vi "Lavi_Ariel_soundboard.vi"() -> ()   [LabVIEW 2016]
uses:
  <vilib>/sound2/lvsound2.llb/Sound Data Format.ctl
  <vilib>/sound2/lvsound2.llb/Sampling Mode.ctl
  <vilib>/sound2/lvsound2.llb/Sound File Position.ctl
  <vilib>/sound2/lvsound2.llb/Sound File Write Open.vi
  <vilib>/sound2/lvsound2.llb/Sound Input Read (DBL).vi
  <vilib>/sound2/lvsound2.llb/Sound File Write (DBL).vi
  <vilib>/sound2/lvsound2.llb/Sound File Info (path).vi
  <vilib>/sound2/lvsound2.llb/Sound File Read Open.vi
  <vilib>/sound2/lvsound2.llb/Sound File Read (DBL).vi
  <vilib>/sound2/lvsound2.llb/Sound Output Set Volume (Single).vi
  <vilib>/sound2/lvsound2.llb/Sound Output Write (DBL).vi
  <vilib>/measure/maspectr.llb/FFT Power Spectrum and PSD for 1 Chan.vi
  <vilib>/measure/NI_MAPro.lvlib
panel:
  in  "Volume":dbl(knob)=100.0 scale=0.0..100.0
  in  "Record start":bool
  in  "Exit":bool
  in  "Menu":bool
  in  "STOP":bool
  in  "Play":bool
  out "f0":dbl
  out "df (increment)":dbl
  out "magnitude":dbl[](array[numeric])
  in  "Playback speed":dbl=1.0
  out "Waveform Graph 2":waveform(dbl)[](graph)
  in  "Upper Cut-Off (Hz)":dbl(slide)=400.0 caption="Upper Cut-Off" scale=20.0..20000.0
  in  "Lower Cut-Off (Hz)":dbl(slide)=100.0 caption="Lower Cut-Off" scale=20.0..20000.0
  in  "Filter enable":bool
  out "Save File path":path
  in  "Pause":bool
  out "Temporary Input File Path":path
  in  "output device ID":u32
  out "Waveform Graph":waveform(dbl)[](graph)
  in  "Record stop":bool
  in  "input device ID":u32
  # "Output Controls/Indicators"
  # "Input Controls/Indicators"
  # "Playback Controls"
  # "NOTE: The \"Menu\" button always\nreturns the user to the last main \nmenu. The \"Exit\" button always\ncauses the VI to stop and close."
  # "Fourier Analysis"
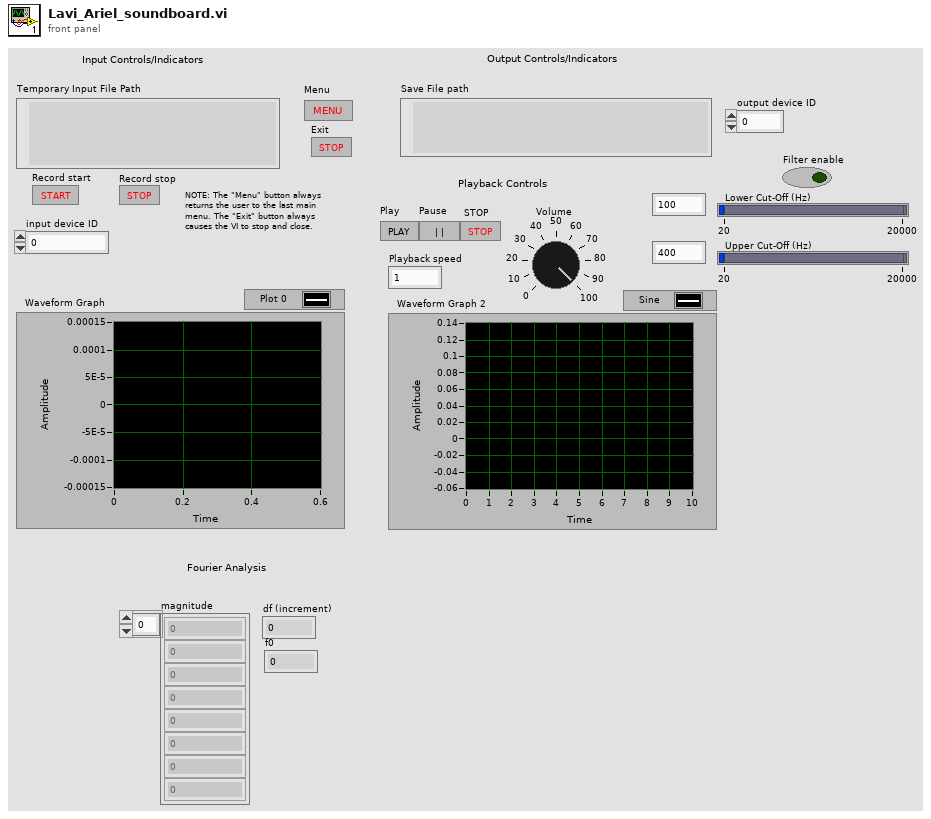
[diagram p1: front panel]
types:
  T1 = typedef "Sampling Mode.ctl" = i32
  T2 = typedef "Sound Data Format.ctl" = cluster{"sample rate (S/s)":dbl, "number of channels":i32, "bits per sample":i32}
  T3 = typedef "Sound File Refnum.ctl" = refnum<file>
  T4 = typedef "Sound Input Task ID.ctl" = u32
  T5 = cluster{dbl, "number of channels":i32, "bits per sample":i32}
  T6 = typedef "Sound Output Task ID.ctl" = u32
  T7 = typedef "Sound File Position.ctl" = u16
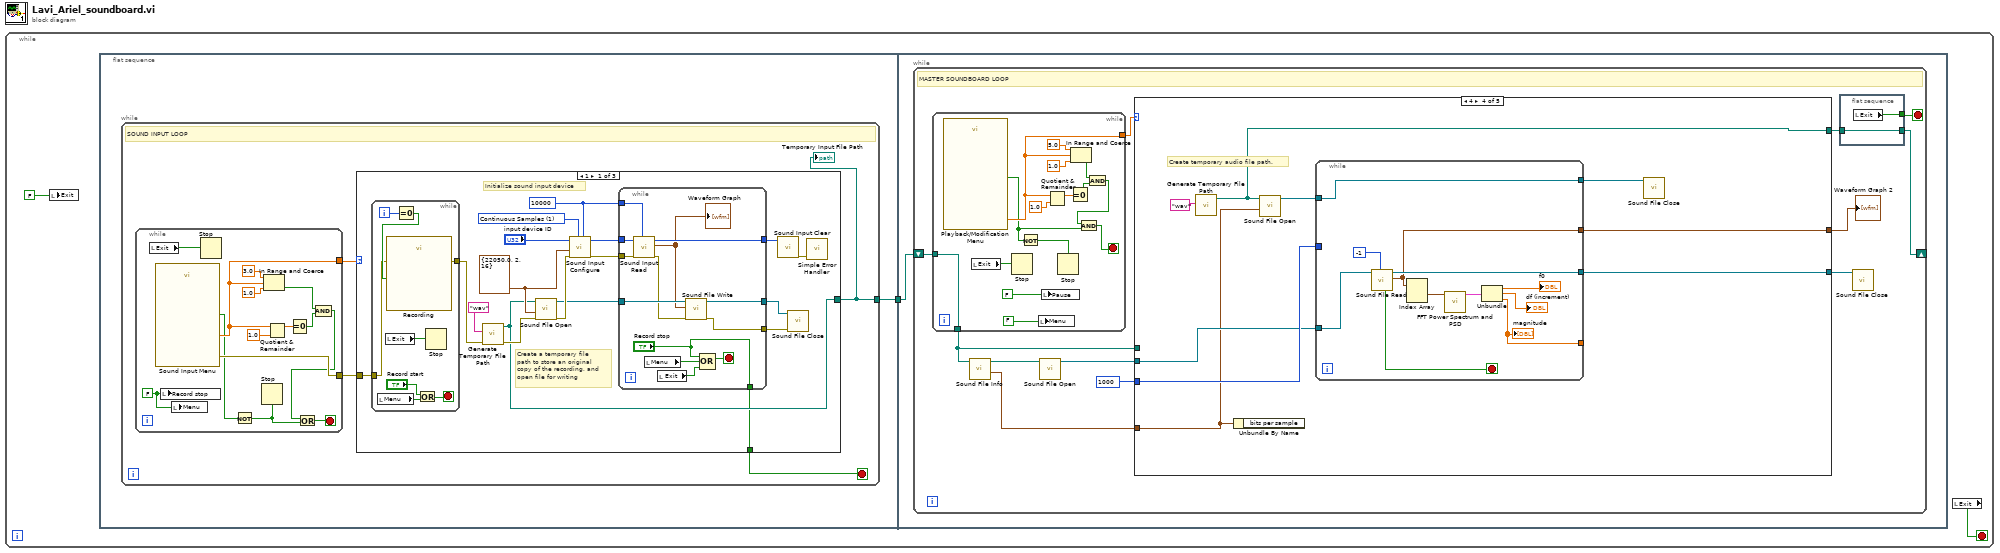
[diagram p0: block diagram]
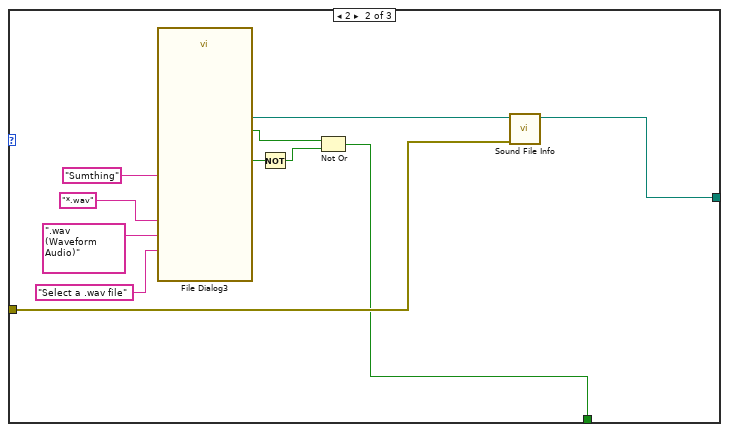
[diagram p2: hidden frame]
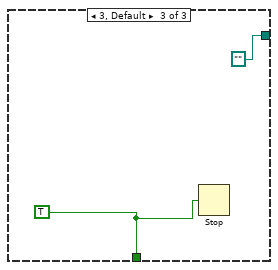
[diagram p3: hidden frame]
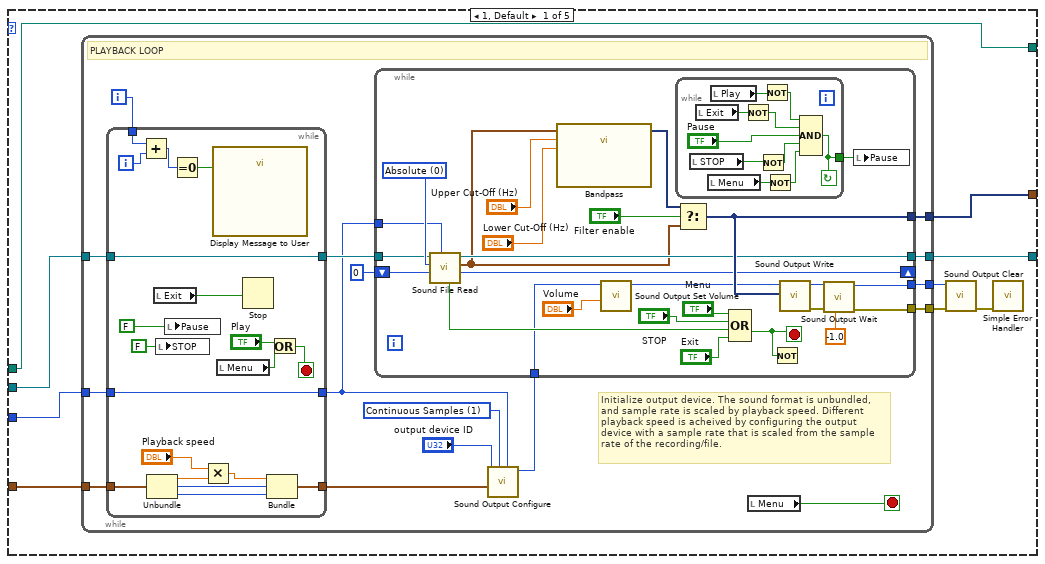
[diagram p4: hidden frame]
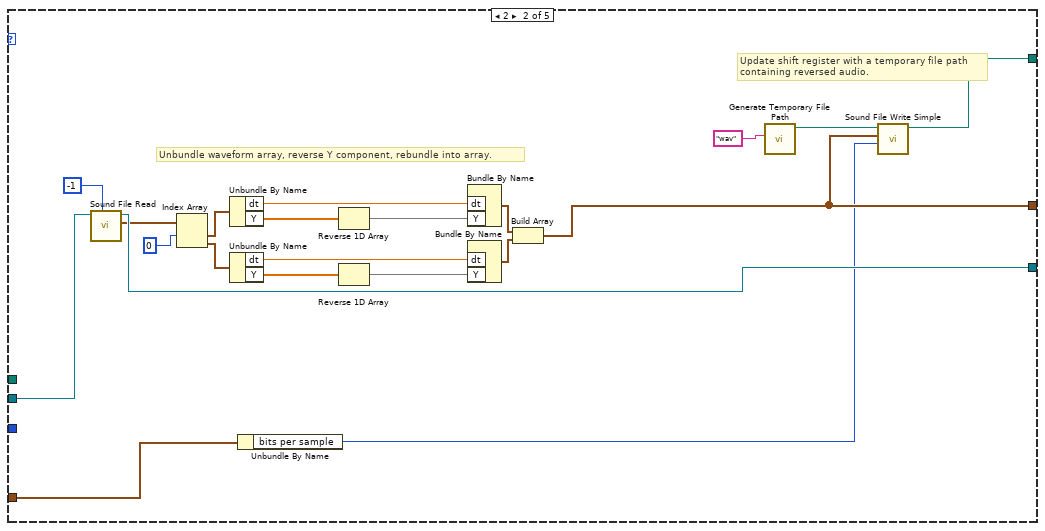
[diagram p5: hidden frame]
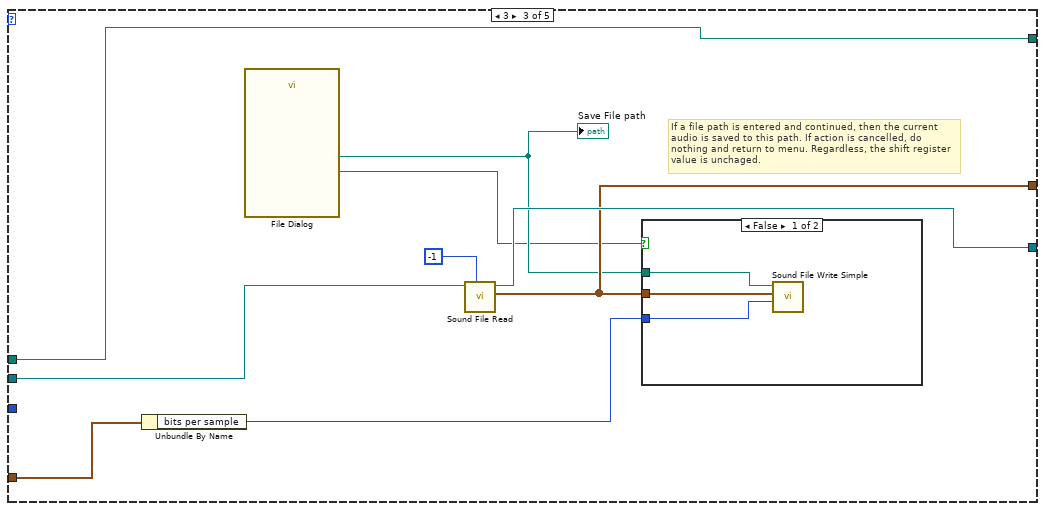
[diagram p6: hidden frame]
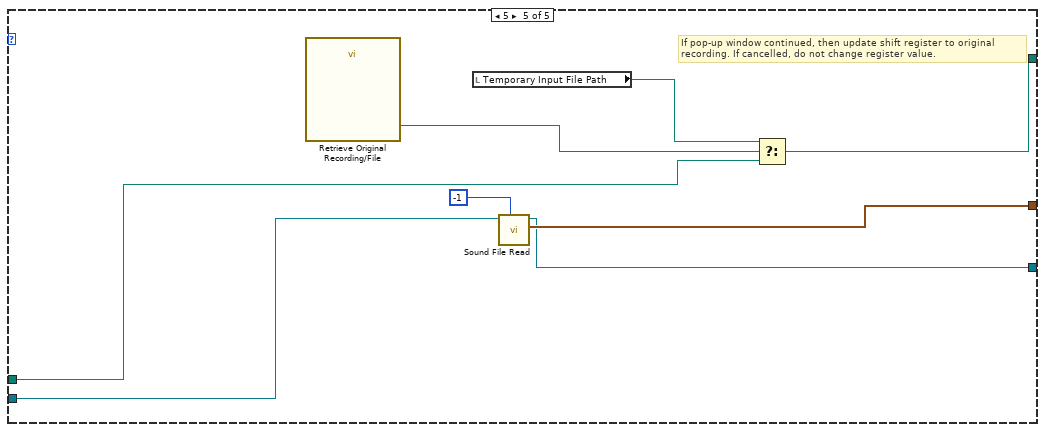
[diagram p8: hidden frame]
diagram:
  n1 = while {
    stop <- w1 stop-if-true
    n2 = local write "Exit"(FALSE) -> ()
    n3 = flat-sequence {
      tunnel: [w4] -> w3
      tunnel: w3 -> [w75]
      frame #0 {
        n4 = while "Input Loop" {
          tunnel: [w5] -> w4
          stop <- w6 stop-if-true
          # "SOUND INPUT LOOP"
          n5 = while {
            tunnel: [w22] -> w8
            tunnel: [w15] -> w7
            stop <- w13 stop-if-true
            w10 = FALSE ("Record stop")
            n6 = local read "Exit"() -> (w9:bool)
            n7 = call "Sound Input Menu"() -> ("Select 1-3"=w15:dbl, "Continue"=w12:bool, "error out"=w22:errorcluster)  [unwired: 17 in]
            n8 = local write "Record stop"(w10) -> ()
            n9 = local write "Menu"(w10) -> ()
            n10 = Stop(stop? (T)=w9) -> ()
            n11 = Not(x=w12) -> (.not. x?=w11:bool)
            n12 = Stop(stop? (T)=w11) -> ()
            n13 = In Range and Coerce(upper limit=3.0 ("lower limit"), x=w15, lower limit=1.0) -> (In Range?=w18:bool)  [unwired: 1 out]
            n14 = Quotient & Remainder(x=w15, y=1.0) -> (x-y*floor(x/y)=w20:dbl)  [unwired: 1 out]
            n15 = Equal To 0?(x=w20) -> (x = 0?=w19:bool)
            n16 = Compound Arithmetic op=AND(w18, w19) -> (w14:bool)
            n17 = Or(x=w14, y=w11) -> (x .or. y?=w13:bool)
          }
          n18 = case shown="1" w7 {
            tunnel: [w27 w67 path ""] -> w5
            tunnel: w8 -> [w24 w72 _]
            tunnel: [w26 w65 w73] -> w6
            frame 1 {
              w28 = 10000 ("number of samples/ch")
              w39 = T1 1 items=["Finite Samples", "Continuous Samples"] ("sample mode")
              w32 = T2 {"sample rate (S/s)"=22050.0, "number of channels"=2, "bits per sample"=16} ("sound format")
              # "Create a temporary file path to store an original copy of the recording, and open file for writing"
              # "Initialize sound input device"
              n19 = while {
                tunnel: w24 -> [w46]
                tunnel: [w45] -> w23
                i -> [w48]
                stop <- w43 stop-if-true
                n20 = local read "Menu"() -> (w41:bool)
                n21 = local read "Exit"() -> (w44:bool)
                n22 = Equal To 0?(x=w48) -> (x = 0?=w47:bool)
                n23 = call "Recording"("error in (no error)"=w46, "Enable"=w47) -> ("error out"=w45:errorcluster)  [unwired: 8 in, 1 out]
                n24 = Or(x="Record start", y=w41) -> (x .or. y?=w43:bool)
                n25 = Stop(stop? (T)=w44) -> ()
              }
              n26 = call <vilib>:"Generate Temporary File Path.vi"("error in (no error)"=w23, "Temporary File Extension (tmp)"="wav") -> ("error out"=w35:errorcluster, "Unique Temporary File Path"=w27:path)  [unwired: 8 in]
              n27 = call-poly <vilib>:"Sound File Open.vi"("error in (no error)"=w35, "sound format"=w32, "path"=w27) -> ("error out"=w36:errorcluster, "sound file refnum"=w33:T3)  [unwired: 7 in]
              n28 = call <vilib>:"Sound Input Configure.vi"("number of samples/ch"=w28, "sample mode"=w39, "error in (no error)"=w36, "sound format"=w32, "device ID"="input device ID") -> ("error out"=w37:errorcluster, "task ID"=w30:T4)  [unwired: 5 in]
              n29 = while {
                tunnel: w30 -> [w61]
                tunnel: w28 -> [w60]
                tunnel: [w59] -> w34
                tunnel: w33 -> [w58]
                tunnel: [w57] -> w40
                tunnel: w37 -> [w56]
                tunnel: [w54] -> w25
                tunnel: ["Record stop"] -> w26
                stop <- w53 stop-if-true
                n30 = call-poly <vilib>:"Sound Input Read.vi"("number of samples/ch"=w60, "error in (no error)"=w56, "task ID"=w61) -> ("error out"=w55:errorcluster, "data"=w49:waveform(dbl)[], "task ID out"=w59:T4)  [unwired: 6 in]
                "Waveform Graph" <- w49
                n31 = local read "Menu"() -> (w52:bool)
                n32 = local read "Exit"() -> (w50:bool)
                n33 = call-poly <vilib>:"Sound File Write.vi"("error in (no error)"=w55, "data"=w49, "sound file refnum"=w58) -> ("error out"=w54:errorcluster, "sound file refnum out"=w57:T3)  [unwired: 7 in]
                n34 = Compound Arithmetic op=OR("Record stop", w52, w50) -> (w53:bool)
              }
              n35 = call <vilib>:"Sound Input Clear.vi"("task ID"=w34) -> ("error out"=w38:errorcluster)  [unwired: 10 in]
              n36 = call <vilib>:"Sound File Close.vi"("error in (no error)"=w25, "sound file refnum"=w40) -> ()  [unwired: 9 in, 1 out]
              n37 = call <vilib>:"Simple Error Handler.vi"("error in (no error)"=w38) -> ()  [unwired: 4 in, 5 out]
            }
            frame 2 {
              n38 = call "File Dialog3"("prompt"="Select a .wav file", "button label"="Sumthing", "pattern (all files)"="*.wav", "pattern label"=".wav (Waveform Audio)" ("pattern (all files)")) -> ("selected path"=w71:path, "exists"=w69:bool, "cancelled"=w70:bool)  [unwired: 8 in, 1 out]
              n39 = Not(x=w69) -> (.not. x?=w68:bool)
              n40 = Not Or(1:w68, 2:w70) -> (0:w65:bool)
              n41 = call-poly <vilib>:"Sound File Info.vi"("error in (no error)"=w72, "path"=w71) -> ("path out"=w67:path)  [unwired: 6 in, 3 out]
            }
            frame 3, Default {
              w73 = TRUE
              n42 = Stop(stop? (T)=w73) -> ()
            }
          }
          "Temporary Input File Path" <- w5
        }
      }
      frame #1 {
        n43 = while {
          shift-right: [w77] -> _
          shift-left: w75 -> [w81]
          stop <- w76 stop-if-true
          # "MASTER SOUNDBOARD LOOP"
          n44 = while {
            tunnel: [w96] -> w84
            tunnel: w81 -> [w93]
            tunnel: [w93] -> w80
            stop <- w98 stop-if-true
            n45 = call "Playback/Modification Menu"() -> ("Select 1-5"=w96:dbl, "Continue"=w94:bool)  [unwired: 17 in, 1 out]
            n46 = local read "Exit"() -> (w90:bool)
            n47 = Stop(stop? (T)=w90) -> ()
            n48 = Not(x=w94) -> (.not. x?=w95:bool)
            n49 = local write "Menu"(FALSE ("Menu")) -> ()
            n50 = local write "Pause"(FALSE ("Playback stop")) -> ()
            n51 = Quotient & Remainder(x=w96, y=1.0) -> (x-y*floor(x/y)=w102:dbl)  [unwired: 1 out]
            n52 = Stop(stop? (T)=w95) -> ()
            n53 = Equal To 0?(x=w102) -> (x = 0?=w100:bool)
            n54 = In Range and Coerce(upper limit=5.0 ("lower limit"), x=w96, lower limit=1.0) -> (In Range?=w101:bool)  [unwired: 1 out]
            n55 = And(x=w101, y=w100) -> (x .and. y?=w99:bool)
            n56 = And(x=w99, y=w94) -> (x .and. y?=w98:bool)
          }
          n57 = call-poly <vilib>:"Sound File Info.vi"("path"=w80) -> ("sound format"=w83:T2, "path out"=w85:path)  [unwired: 7 in, 2 out]
          n58 = call-poly <vilib>:"Sound File Open.vi"("path"=w85) -> ("sound file refnum"=w86:T3)  [unwired: 9 in, 1 out]
          n59 = case shown="4" w84 {
            tunnel: [w109 w204 w213 w225 w243] -> w87
            tunnel: w86 -> [w105 w205 w214 w224 w244]
            tunnel: u32 1000 ("Samples/iteration") -> [w106 _ _ w226 _]
            tunnel: w83 -> [w107 w188 w211 w221 _]
            tunnel: [w113 w190 w212 w222 w245] -> w82
            tunnel: [w112 w186 w207 w219 w239] -> w78
            tunnel: w80 -> [w112 _ w207 _ w240]
            frame 1, Default {
              n60 = while {
                tunnel: [w123] -> w110
                tunnel: [w129] -> w113
                tunnel: [w126] -> w109
                tunnel: [w122] -> w108
                tunnel: w106 -> [w118]
                tunnel: w107 -> [w121]
                tunnel: w105 -> [w120]
                i -> [w114]
                stop <- w115 stop-if-true
                w128 = T1 1 items=["Finite Samples", "Continuous Samples"] ("sample mode")
                # "Initialize output device. The sound format is unbundled, and sample rate is scaled by playback speed. Different playback speed is acheived by configuring the output device with a sample rate that is scaled from the sample rate of the recording/file."
                # "PLAYBACK LOOP"
                n61 = while {
                  tunnel: w121 -> [w141]
                  tunnel: [w139] -> w116
                  tunnel: w120 -> [w137]
                  tunnel: [w137] -> w119
                  tunnel: [w136] -> w117
                  tunnel: w118 -> [w136]
                  tunnel: w114 -> [w135]
                  i -> [w134]
                  stop <- w130 stop-if-true
                  n62 = Add(x=w135, y=w134) -> (x+y=w133:i32)
                  n63 = Unbundle(w141) -> ("sample rate (S/s)"=w140:dbl, "number of channels"=w143:i32, "bits per sample"=w142:i32)
                  n64 = local read "Exit"() -> (w138:bool)
                  n65 = local write "STOP"(FALSE ("STOP")) -> ()
                  n66 = local write "Pause"(FALSE ("Playback stop")) -> ()
                  n67 = Equal To 0?(x=w133) -> (x = 0?=w147:bool)
                  n68 = Multiply(x="Playback speed", y=w140) -> (x*y=w144:dbl)
                  n69 = call "Display Message to User"("Enable"=w147) -> ()  [unwired: 9 in, 2 out]
                  n70 = local read "Menu"() -> (w131:bool)
                  n71 = Stop(stop? (T)=w138) -> ()
                  n72 = Bundle(w144, "number of channels"=w143, "bits per sample"=w142) -> (w139:T5)  [unwired: 1 in]
                  n73 = Or(x="Play", y=w131) -> (x .or. y?=w130:bool)
                }
                n74 = call <vilib>:"Sound Output Configure.vi"("number of samples/ch"=w117, "sample mode"=w128, "sound format"=w116, "device ID"="output device ID") -> ("task ID"=w125:T6)  [unwired: 6 in, 1 out]
                n75 = while {
                  tunnel: [w162] -> w123
                  tunnel: [w170] -> w129
                  tunnel: [w161] -> w122
                  tunnel: [w169] -> w126
                  tunnel: w125 -> [w150]
                  shift-right: [w165] -> _
                  shift-left: 0 ("offset") -> [w166]
                  tunnel: w119 -> [w156]
                  tunnel: w117 -> [w155]
                  stop <- w157 stop-if-true
                  w167 = T7 0 items=["Absolute"=0, "Relative"=2] ("position mode")
                  n76 = call-poly <vilib>:"Sound File Read.vi"("number of samples/ch (-1: all)"=w155, "position offset"=w166, "position mode"=w167, "sound file refnum"=w156) -> ("offset"=w165:i32, "data"=w168:waveform(dbl)[], "sound file refnum out"=w169:T3, "end of file?"=w158:bool)  [unwired: 3 in, 1 out]
                  n77 = call "Bandpass"("Lower Cut-Off"="Lower Cut-Off (Hz)", "Upper Cut-Off"="Upper Cut-Off (Hz)", "Signal"=w168) -> ("Filtered Signal"=w171:dynamicdata)  [unwired: 7 in, 1 out]
                  n78 = call-poly <vilib>:"Sound Output Set Volume.vi"("volume"="Volume", "task ID"=w150) -> ("task ID out"=w151:T6)  [unwired: 8 in, 1 out]
                  n79 = while {
                    tunnel: [w175] -> w152
                    stop <- w175 continue-if-true
                    n80 = local read "STOP"() -> (w182:bool)
                    n81 = local read "Exit"() -> (w177:bool)
                    n82 = local read "Menu"() -> (w181:bool)
                    n83 = local read "Play"() -> (w179:bool)
                    n84 = Not(x=w177) -> (.not. x?=w176:bool)
                    n85 = Not(x=w182) -> (.not. x?=w183:bool)
                    n86 = Not(x=w179) -> (.not. x?=w178:bool)
                    n87 = Not(x=w181) -> (.not. x?=w180:bool)
                    n88 = Compound Arithmetic op=AND(w178, w176, "Pause", w183, w180) -> (w175:bool)
                  }
                  n89 = Select(t=w171, s="Filter enable", f=w168) -> (s? t:f=w170:dynamicdata)
                  n90 = Compound Arithmetic op=OR("Menu", "STOP", w158, "Exit") -> (w157:bool)
                  n91 = Not(x=w157) -> ()  [unwired: 1 out]
                  n92 = call-poly <vilib>:"Sound Output Write.vi"("data"=w170, "task ID"=w151) -> ("error out"=w164:errorcluster, "task ID out"=w163:T6)  [unwired: 8 in]
                  n93 = call <vilib>:"Sound Output Wait.vi"("timeout (sec)"=-1.0, "error in (no error)"=w164, "task ID"=w163) -> ("error out"=w161:errorcluster, "task ID out"=w162:T6)  [unwired: 7 in]
                  n94 = local write "Pause"(w152) -> ()
                }
                n95 = local read "Menu"() -> (w115:bool)
              }
              n96 = call <vilib>:"Sound Output Clear.vi"("error in (no error)"=w108, "task ID"=w110) -> ("error out"=w111:errorcluster)  [unwired: 9 in]
              n97 = call <vilib>:"Simple Error Handler.vi"("error in (no error)"=w111) -> ()  [unwired: 4 in, 5 out]
            }
            frame 2 {
              # "Update shift register with a temporary file path\ncontaining reversed audio."
              # "Unbundle waveform array, reverse Y component, rebundle into array."
              n98 = call-poly <vilib>:"Sound File Read.vi"("number of samples/ch (-1: all)"=-1, "sound file refnum"=w205) -> ("data"=w201:waveform(dbl)[], "sound file refnum out"=w204:T3)  [unwired: 5 in, 3 out]
              n99 = Index Array(array=w201, index #1=0 ("index")) -> (element #1=w202:waveform(dbl), element #2=w200:waveform(dbl))  [unwired: 1 in]
              n100 = Unbundle By Name(w202) -> ("dt"=w197:dbl, "Y"=w199:dbl[])
              n101 = Unbundle By Name(w200) -> ("dt"=w196:dbl, "Y"=w198:dbl[])
              n102 = Unbundle By Name(w188) -> ("bits per sample"=w187:i32)
              n103 = Reverse 1D Array(array=w199) -> (reversed array=w195:dbl[])
              n104 = Reverse 1D Array(array=w198) -> (reversed array=w194:dbl[])
              n105 = Bundle By Name("dt"=w197, "Y"=w195) -> (w193:waveform(dbl))  [unwired: 1 in]
              n106 = Bundle By Name("dt"=w196, "Y"=w194) -> (w192:waveform(dbl))  [unwired: 1 in]
              n107 = Build Array(w193, w192) -> (w190:waveform(dbl)[])
              n108 = call <vilib>:"Generate Temporary File Path.vi"("Temporary File Extension (tmp)"="wav") -> ("Unique Temporary File Path"=w189:path)  [unwired: 9 in, 1 out]
              n109 = call <vilib>:"Sound File Write Simple.vi"("bits per sample"=w187, "data"=w190, "path"=w189) -> ("path out"=w186:path)  [unwired: 7 in, 1 out]
            }
            frame 3 {
              # "If a file path is entered and continued, then the current\naudio is saved to this path. If action is cancelled, do nothing and return to menu. Regardless, the shift register value is unchaged."
              n110 = Unbundle By Name(w211) -> ("bits per sample"=w210:i32)
              n111 = call "File Dialog"() -> ("selected path"=w209:path, "cancelled"=w208:bool)  [unwired: 12 in, 2 out]
              "Save File path" <- w209
              n112 = call-poly <vilib>:"Sound File Read.vi"("number of samples/ch (-1: all)"=-1, "sound file refnum"=w214) -> ("data"=w212:waveform(dbl)[], "sound file refnum out"=w213:T3)  [unwired: 5 in, 3 out]
              n113 = case shown="False" w208 {
                tunnel: w212 -> [w217 _]
                tunnel: w210 -> [w216 _]
                tunnel: w209 -> [w215 _]
                frame False {
                  n114 = call <vilib>:"Sound File Write Simple.vi"("bits per sample"=w216, "data"=w217, "path"=w215) -> ()  [unwired: 7 in, 2 out]
                }
                frame True {
                }
              }
            }
            frame 4 {
              # "Create temporary audio file path."
              n115 = call <vilib>:"Generate Temporary File Path.vi"("Temporary File Extension (tmp)"="wav") -> ("Unique Temporary File Path"=w219:path)  [unwired: 9 in, 1 out]
              n116 = Unbundle By Name(w221) -> ()  [unwired: 1 out]
              n117 = call-poly <vilib>:"Sound File Open.vi"("sound format"=w221, "path"=w219) -> ("sound file refnum"=w220:T3)  [unwired: 8 in, 1 out]
              n118 = while {
                tunnel: w226 -> [_]
                tunnel: w224 -> [w236]
                tunnel: [w237] -> w225
                tunnel: [w233] -> w222
                tunnel: w220 -> [w229]
                tunnel: [w229] -> w218
                tunnel: [w227] -> _
                stop <- w235 stop-if-true
                n119 = call-poly <vilib>:"Sound File Read.vi"("number of samples/ch (-1: all)"=-1, "sound file refnum"=w236) -> ("data"=w233:waveform(dbl)[], "sound file refnum out"=w237:T3, "end of file?"=w235:bool)  [unwired: 5 in, 2 out]
                n120 = Index Array(array=w233) -> (element #1=w232:waveform(dbl))  [unwired: 2 in, 1 out]
                n121 = call-poly <vilib>:"FFT Power Spectrum and PSD.vi"("time signal"=w232) -> ("Power Spectrum / PSD"=w234:cluster{"f0":dbl, "df":dbl, "magnitude":dbl[]})  [unwired: 7 in, 3 out]
                n122 = Unbundle(w234) -> ("f0"=→"f0":dbl, "df"=→"df (increment)":dbl, "magnitude"=w227:dbl[])
                "magnitude" <- w227
              }
              n123 = call <vilib>:"Sound File Close.vi"("sound file refnum"=w218) -> ()  [unwired: 10 in, 1 out]
            }
            frame 5 {
              # "If pop-up window continued, then update shift register to original\nrecording. If cancelled, do not change register value."
              n124 = call "Retrieve Original Recording/File"() -> ("Continue"=w242:bool)  [unwired: 18 in, 1 out]
              n125 = local read "Temporary Input File Path"() -> (w241:path)
              n126 = call-poly <vilib>:"Sound File Read.vi"("number of samples/ch (-1: all)"=-1, "sound file refnum"=w244) -> ("data"=w245:waveform(dbl)[], "sound file refnum out"=w243:T3)  [unwired: 5 in, 3 out]
              n127 = Select(t=w241, s=w242, f=w240) -> (s? t:f=w239:path)
            }
          }
          "Waveform Graph 2" <- w82
          n128 = flat-sequence {
            tunnel: [w88] -> w76
            tunnel: w78 -> [w89]
            tunnel: [w89] -> w77
            frame #0 {
              n129 = local read "Exit"() -> (w88:bool)
            }
          }
          n130 = call <vilib>:"Sound File Close.vi"("sound file refnum"=w87) -> ()  [unwired: 10 in, 1 out]
        }
      }
    }
    n131 = local read "Exit"() -> (w1:bool)
  }
